vi "StringToArrays.vi"(0 "String":string, 1 "Deliminator":string=",") -> (2 "StringArr":string[](array[string]), 3 "DblArr":dbl[](array[numeric]) format="%.2f", 4 "I32Arr":i32[](array[numeric]))   [LabVIEW 2011]
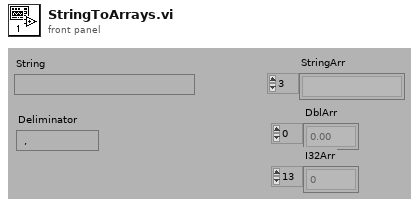
[diagram p1: front panel]
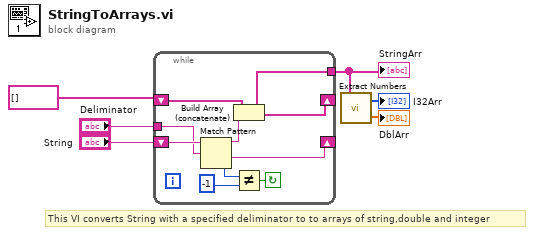
[diagram p0: block diagram]
diagram:
  # "This VI converts String with a specified deliminator to to arrays of string,double and integer"
  n1 = while {
    shift-right: [w10] -> _
    shift-left: "String" -> [w15]
    shift-right: [w8] -> _
    shift-left: string[] [] -> [w11]
    tunnel: [w8] -> w5
    tunnel: "Deliminator" -> [w7]
    stop <- w12 continue-if-true
    n2 = Match Pattern(string=w15, regular expression=w7) -> (before substring=w9:string, after substring=w10:string, offset past match=w13:i32)  [unwired: 1 in, 1 out]
    n3 = Build Array (concatenate)(w11, w9) -> (w8:string[])
    n4 = Not Equal?(x=w13, y=-1) -> (x != y?=w12:bool)
  }
  "StringArr" <- w5
  n5 = call "Extract Numbers.vi"("Strimg[]"=w5) -> ("I32[]"=→"I32Arr":i32[], "Sgl[]"=→"DblArr":dbl[])
